vi "Actor Core.vi"(8 "error in":errorcluster, 11 "Cooler UI":refnum<class "Programmatic Controller.lvclass">) -> (0 "error out":errorcluster, 3 "Actor out":refnum<class "Actor.lvclass">)   [LabVIEW 2018, in "Programmatic Controller.lvclass"]
doc: "This is Actor Core.vi, the main message handling loop for Actors. An actor usually just sits in this loop and processes messages as they arrive. Any error returned by the message Do.vi call will stop the loop, with error code 43 as the canonical signal to stop with no error sent to caller. Descendants may override that in Handle Error.vi."
uses:
  Programmatic Controller.lvclass
  C:/GitClones/LGP5-Resources/Frameworks/Actor Framework/Feedback Evaporative Cooler/Cooler Controller/Cooler Controller/Cooler Controller.lvclass
  C:/Program Files (x86)/National Instruments/LabVIEW 2018/vi.lib/ActorFramework/Actor/Actor.lvclass
  <vilib>/ActorFramework/Actor/Actor.lvclass
  <vilib>/ActorFramework/Actor/Actor.lvclass/Actor.ctl
  <vilib>/ActorFramework/Message Enqueuer/Message Enqueuer.lvclass/Message Enqueuer.ctl
  Air Cooler Application/Load Into Sub Panel Msg/Load Into Sub Panel Msg.lvclass/Load Into Sub Panel Msg.ctl
  Programmatic Controller.lvclass/Programmatic Controller.ctl
  Cooler Controller/Change Desired Temperature Msg/Change Desired Temperature Msg.lvclass/Change Desired Temperature Msg.ctl
  <vilib>/ActorFramework/Message Enqueuer/Init from Existing Queue.vi
  <vilib>/ActorFramework/Message Enqueuer/Enqueue.vi
  Air Cooler Application/Load Into Sub Panel Msg/Load Into Sub Panel Msg.lvclass
  C:/Program Files (x86)/National Instruments/LabVIEW 2018/vi.lib/ActorFramework/Message/Message.lvclass
  <vilib>/ActorFramework/Stop Msg/Stop Msg.lvclass
  Cooler Controller/Change Desired Temperature Msg/Change Desired Temperature Msg.lvclass
  <vilib>/ActorFramework/Message Priority Queue/Priority Enqueue.vi
  <vilib>/ActorFramework/Message Enqueuer/Message Enqueuer.lvclass
  Cooler Controller/Cooler Controller/Cooler Controller.lvclass
panel:
  in  "Time Display":string="%1.2f seconds"
  out "Time Elapsed":string
  out "Programmed Sequence":enum32{"Step 1", "Step 2", "Step 3", "Step 4"}(radio)
  out "Event Log":string
  in  "stop":bool
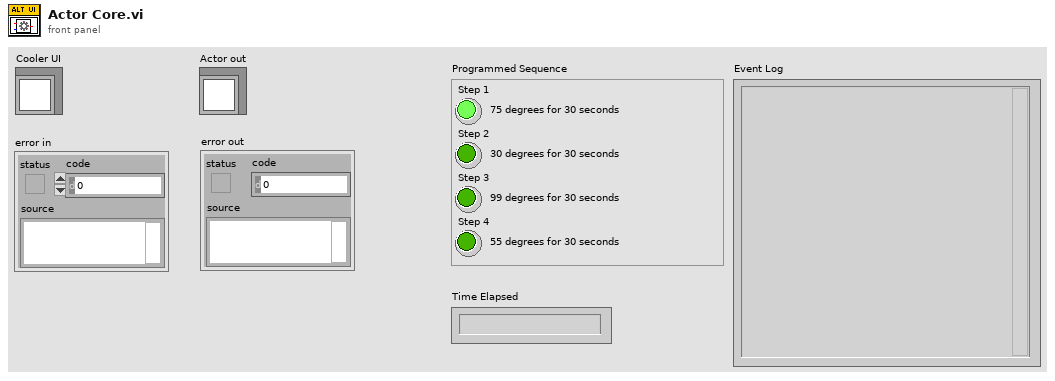
[diagram p1: front panel]
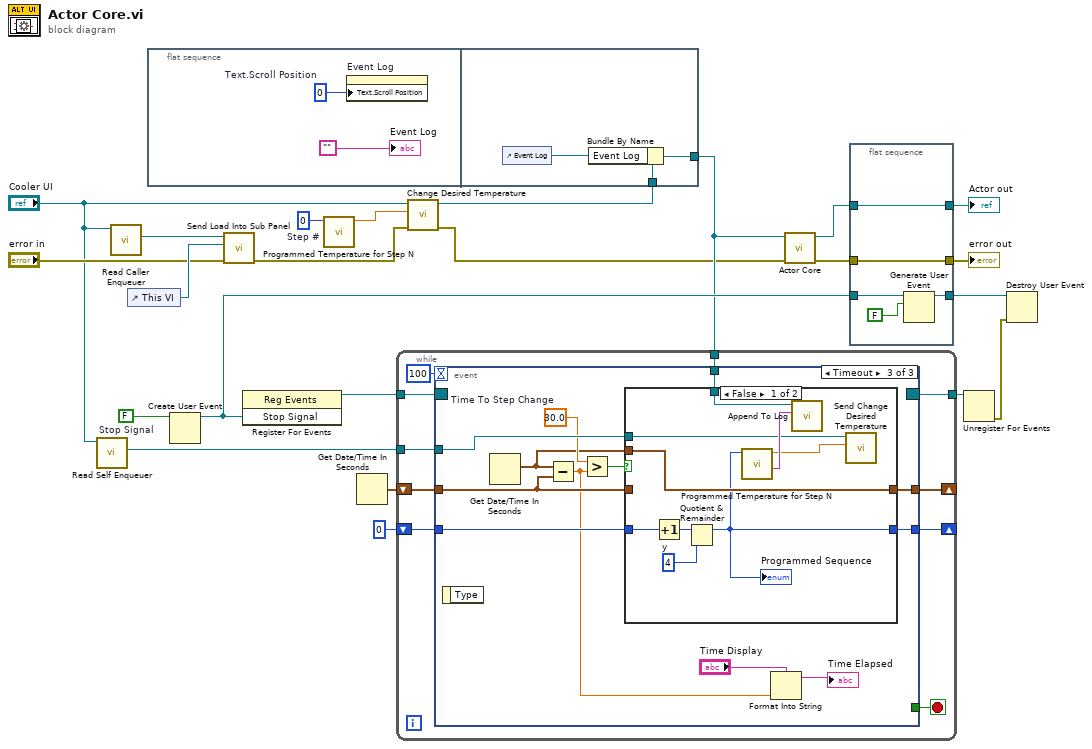
[diagram p0: block diagram]
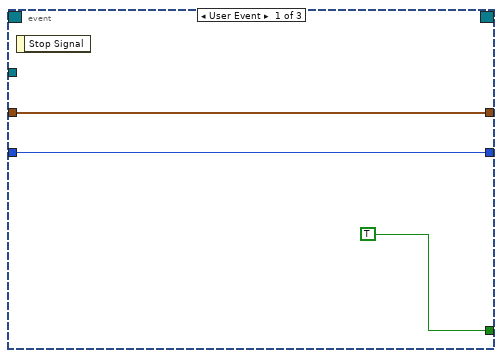
[diagram p2: hidden frame]
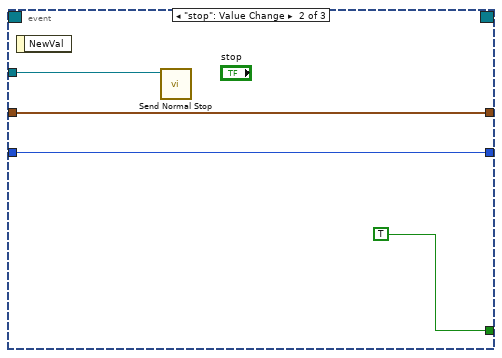
[diagram p3: hidden frame]
diagram:
  w8 = 0  # Step #
  w15 = FALSE  # Stop Signal
  n1 = call <vilib>:"Read Self Enqueuer.vi"("Actor"="Cooler UI") -> ("Self Enqueuer"=w6:refnum<class "Message Enqueuer.lvclass">)  [unwired: 10 in]
  n2 = call <vilib>:"Read Caller Enqueuer.vi"("Actor"="Cooler UI") -> ("Caller Enqueuer"=w13:refnum<class "Message Enqueuer.lvclass">)  [unwired: 10 in]
  n3 = control-ref of="This VI"() -> (w12:refnum<vi>)
  n4 = flat-sequence {
    tunnel: w4 -> [w28]
    tunnel: [w26] -> w7
    frame #0 {
      w25 = u32 0  # Text.Scroll Position
      n5 = property on="Event Log" class="Str"("Text.Scroll Position"=w25) -> ()  [unwired: 2 in, 2 out]
      "Event Log" <- ""
    }
    frame #1 {
      n6 = control-ref of="Event Log"() -> (w27:refnum<vi>)
      n7 = Bundle By Name(cluster=w28, "Event Log"=w27) -> (w26:refnum<class "Programmatic Controller.lvclass">)
    }
  }
  n8 = Create User Event(user event datatype=w15) -> (user event=w20:refnum<user-event>)  [unwired: 1 in, 1 out]
  n9 = call "Send Load Into Sub Panel.vi"("error in (no error)"="error in", "VI for SubPanel"=w12, "Message Enqueuer"=w13) -> ("error out"=w2:errorcluster)  [unwired: 8 in]
  n10 = register-events(w20) -> (reference out=w23:refnum<event-registration>)  [unwired: 2 in, 1 out]
  n11 = call "Programmed Temperature for Step N.vi"("Step #"=w8) -> ("Desired Temperature"=w3:dbl)  [unwired: 9 in, 1 out]
  n12 = Get Date/Time In Seconds() -> (seconds since 1Jan1904=w10:timestamp)
  n13 = while {
    tunnel: w23 -> [w38]
    tunnel: [w37] -> w22
    tunnel: w6 -> [w35]
    shift-right: [w34] -> _
    shift-left: w10 -> [w33]
    shift-right: [w31] -> _
    shift-left: 0 -> [w32]
    tunnel: w7 -> [w30]
    stop <- w36 stop-if-true
    n14 = event shown="[2] Timeout" {
      selector: w38 -> [_ _ _]
      dyn-events: [_ _ _] -> w37
      timeout: 100 -> [_ _ _]
      tunnel: [TRUE TRUE _] -> w36
      tunnel: w35 -> [_ w45 w57]
      tunnel: [w39 w42 w53] -> w34
      tunnel: w33 -> [w39 w42 w54]
      tunnel: w32 -> [w40 w43 w51]
      tunnel: [w40 w43 w52] -> w31
      tunnel: w30 -> [_ _ w49]
      event User Event {
        n15 = event-data() -> ()  [unwired: 1 in, 1 out]
      }
      event "stop": Value Change {
        n16 = event-data() -> ()  [unwired: 1 in, 1 out]
        n17 = call <vilib>:"Send Normal Stop.vi"("Message Enqueuer"=w45) -> ()  [unwired: 10 in, 1 out]
      }
      event Timeout {
        w56 = 30.0  # Time To Step Change
        n18 = event-data() -> ()  [unwired: 1 in, 1 out]
        n19 = Get Date/Time In Seconds() -> (seconds since 1Jan1904=w50:timestamp)
        n20 = Subtract(x=w50, y=w54) -> (x-y=w46:dbl)
        n21 = Greater?(x=w56, y=w46) -> (0:w55:bool)
        n22 = case shown="False" w55 {
          tunnel: w57 -> [w59 _]
          tunnel: w54 -> [_ w68]
          tunnel: [w66 w68] -> w53
          tunnel: [w62 w67] -> w52
          tunnel: w51 -> [w65 w67]
          tunnel: w50 -> [w66 _]
          tunnel: w49 -> [w61 _]
          frame False {
            w63 = 4  # y
            n23 = Increment(x=w65) -> (x+1=w64:i32)
            n24 = Quotient & Remainder(x=w64, y=w63) -> (x-y*floor(x/y)=w62:i32)  [unwired: 1 out]
            "Programmed Sequence" <- w62
            n25 = call "Programmed Temperature for Step N.vi"("Step #"=w62) -> ("New Temperature  Message"=w60:string, "Desired Temperature"=w58:dbl)  [unwired: 9 in]
            n26 = call "Append To Log.vi"("String"=w60, "Cooler Alternate UI in"=w61) -> ()  [unwired: 9 in, 1 out]
            n27 = call "Send Change Desired Temperature.vi"("Desired Temperature"=w58, "Message Enqueuer"=w59) -> ()  [unwired: 9 in, 1 out]
          }
          frame True {
          }
        }
        n28 = Format Into String(format string="Time Display", w46) -> (resulting string=→"Time Elapsed":string)  [unwired: 2 in, 1 out]
      }
    }
  }
  n29 = call "Change Desired Temperature.vi"("error in (no error)"=w2, "Desired Temperature"=w3, "Cooler Controller in"="Cooler UI") -> ("error out"=w1:errorcluster, "Cooler Controller out"=w4:refnum<class "Programmatic Controller.lvclass">)  [unwired: 7 in]
  n30 = call-parent "Actor Core.vi"("error in"=w1, "Actor in"=w7) -> ("error out"=w16:errorcluster, "Actor out"=w18:refnum<class "Actor.lvclass">)  [unwired: 8 in]
  n31 = flat-sequence {
    tunnel: [w73] -> w21
    tunnel: w20 -> [w72]
    tunnel: w18 -> [w71]
    tunnel: [w71] -> w19
    tunnel: w16 -> [w70]
    tunnel: [w70] -> w17
    frame #0 {
      n32 = Generate User Event(user event=w72, event data cluster=FALSE) -> (user event out=w73:refnum<user-event>)  [unwired: 2 in, 1 out]
    }
  }
  n33 = Unregister For Events(event registration refnum=w22) -> (error out=w14:errorcluster)  [unwired: 1 in]
  n34 = Destroy User Event(user event=w21, error in=w14) -> ()  [unwired: 1 out]
  "error out" <- w17
  "Actor out" <- w19
